vi "20170509-lecture4-2 prof Login.vi"() -> (2 "Correct":bool)   [LabVIEW 2014]
panel:
  in  "stop":bool
  in  "Password":string
  in  "Username":string
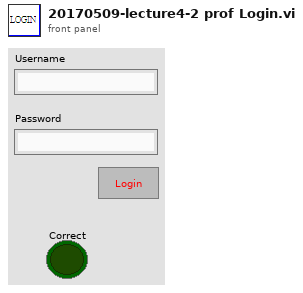
[diagram p1: front panel]
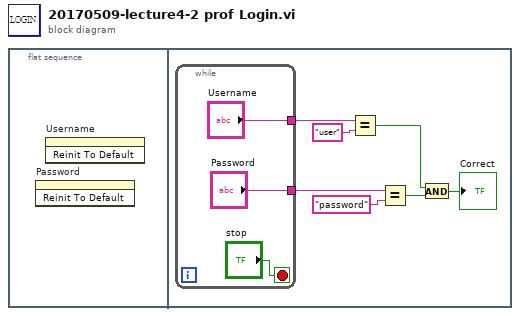
[diagram p0: block diagram]
diagram:
  n1 = flat-sequence {
    frame #0 {
      n2 = invoke on="Password" class="Str" method="Reinit To Default"() -> ()  [unwired: 3 in, 3 out]
      n3 = invoke on="Username" class="Str" method="Reinit To Default"() -> ()  [unwired: 3 in, 3 out]
    }
    frame #1 {
      n4 = while {
        tunnel: ["Username"] -> w2
        tunnel: ["Password"] -> w1
        stop <- "stop" stop-if-true
      }
      n5 = Equal?(x=w2, y="user") -> (x = y?=w5:bool)
      n6 = Equal?(x=w1, y="password") -> (x = y?=w6:bool)
      n7 = And(x=w5, y=w6) -> (x .and. y?=→"Correct":bool)
    }
  }
